vi "AddNewGraph.vi"(8 "error in (no error)":errorcluster caption="entrée d'erreur (pas d'erreur)", 10 "FAIndex":i32=-1, 11 "Interface en entrée":refnum<class "Interface.lvclass"> caption="DNL_LabVIEW Object in") -> (0 "error out":errorcluster caption="sortie d'erreur", 2 "NewGraphInd":i32, 3 "Interface en sortie":refnum<class "Interface.lvclass"> caption="DNL_LabVIEW Object out")   [LabVIEW 2019, in "Interface.lvclass"]
uses:
  Interface.lvclass
  Interface.lvclass/Interface.ctl
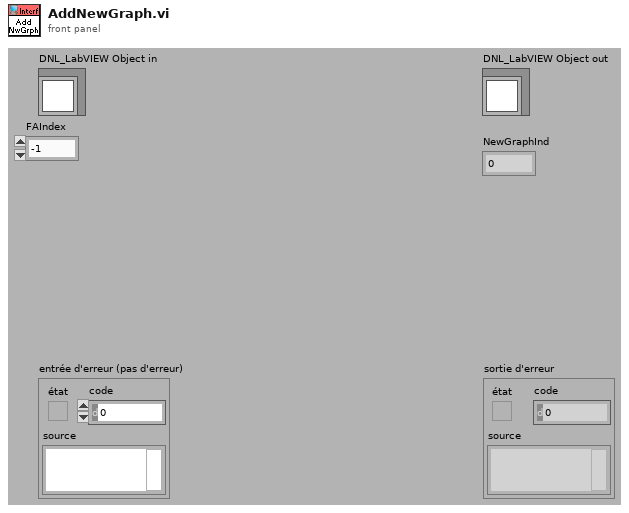
[diagram p1: front panel]
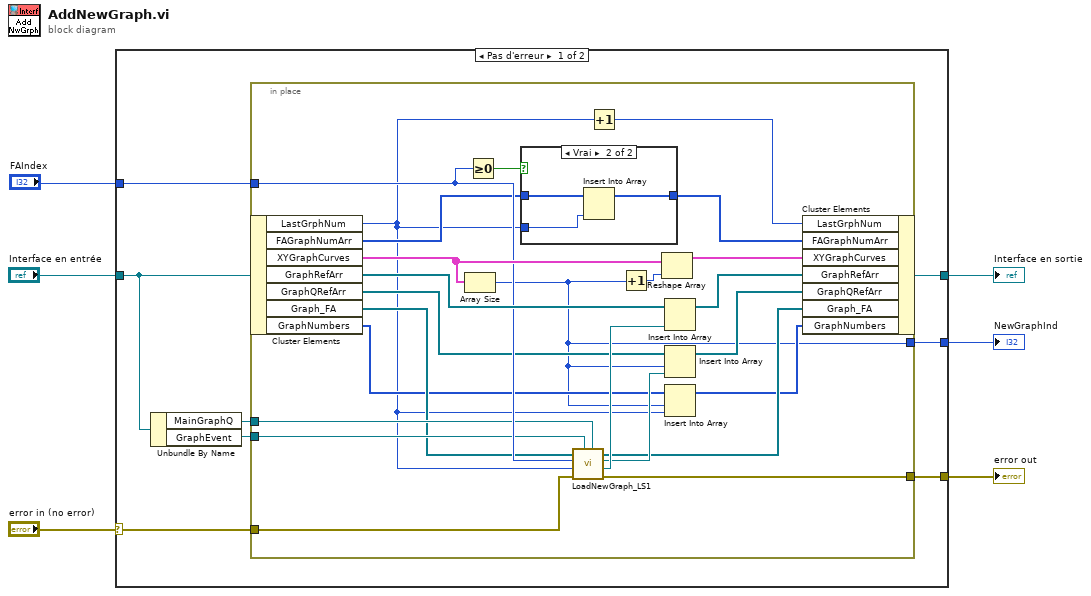
[diagram p0: block diagram]
diagram:
  n1 = case shown="Pas d'erreur" "error in (no error)" {
    selector: "error in (no error)" -> [w7 w44]
    tunnel: [w13 w44] -> w5
    tunnel: [w12 w43] -> w3
    tunnel: "Interface en entrée" -> [w8 w43]
    tunnel: [w14 _] -> w2
    tunnel: "FAIndex" -> [w9 _]
    frame No Error {
      n2 = Unbundle By Name(w8) -> ("MainGraphQ"=w11:refnum<queue>, "GraphEvent"=w10:refnum<user-event>)
      n3 = in-place {
        in-place-border: [w16] -> w14
        in-place-border: w7 -> [w26]
        in-place-border: [w35] -> w13
        in-place-border: w9 -> [w33]
        in-place-border: w11 -> [w25]
        in-place-border: w10 -> [w24]
        n4 = in-place-cluster #1(w8) -> ("LastGrphNum"=w15:i32, "FAGraphNumArr"=w30:i32[], "XYGraphCurves"=w38:cluster{"Tableau":i32[]}[], "GraphRefArr"=w34:refnum<vi>[], "GraphQRefArr"=w21:refnum<queue>[], "Graph_FA"=w23:refnum<vi>[], "GraphNumbers"=w18:i32[])
        n5 = Array Size(array=w38) -> (size(s)=w16:i32)
        n6 = Greater Or Equal To 0?(x=w33) -> (x >= 0?=w32:bool)
        n7 = case shown="Vrai" w32 {
          tunnel: [w39 w42] -> w31
          tunnel: w30 -> [w39 w41]
          tunnel: w15 -> [_ w40]
          frame False {
            # "free floating Graph"
          }
          frame True {
            n8 = Insert Into Array(array=w41, new element=w40) -> (w42:i32[])  [unwired: 1 in]
          }
        }
        n9 = call "LoadNewGraph_LS1.vi"("MainGraphQ"=w25, "GraphEvent"=w24, "ErrIn(No Err)"=w26, "GraphNumber"=w15, "FAIndex"=w33, "Graph_FA"=w23) -> ("ErrOut"=w35:errorcluster, "Graph"=w29:refnum<vi>, "GraphQRef"=w27:refnum<queue>, "Graph_FA Out"=w22:refnum<vi>[])  [unwired: 2 in]
        n10 = Increment(x=w15) -> (x+1=w20:i32)
        n11 = Increment(x=w16) -> (x+1=w37:i32)
        n12 = Reshape Array(w38, w37) -> (w36:cluster{"Tableau":i32[]}[])
        n13 = Insert Into Array(array=w34, new element=w29) -> (w28:refnum<vi>[])  [unwired: 1 in]
        n14 = Insert Into Array(array=w21, index=w16, new element=w27) -> (w19:refnum<queue>[])
        n15 = Insert Into Array(array=w18, index=w16, new element=w15) -> (w17:i32[])
        n16 = in-place-cluster #1("LastGrphNum"=w20, "FAGraphNumArr"=w31, "XYGraphCurves"=w36, "GraphRefArr"=w28, "GraphQRefArr"=w19, "Graph_FA"=w22, "GraphNumbers"=w17) -> (w12:refnum<class "Interface.lvclass">)
      }
    }
    frame Error {
    }
  }
  "error out" <- w5
  "Interface en sortie" <- w3
  "NewGraphInd" <- w2
